vi "Fpga-MicroBlaze-Transmit.vi"(0 "Network API":refnum<class "niInstr Network API FPGA v1.lvclass">, 1 "FIFO In":refnum<k21>, 5 "Controls":T3={"UDP Source Port"=43981, "UDP Destination Port"=61185, "preferred datagram size"=1400, "Use Pattern Gen"=FALSE, "max frame payload"=1472, "minimum packet interval"=1, "stream.num samples 0"=0, "stream.request state 0"=enum."Idle"} {"UDP Destination Port" format="%04x"; "UDP Source Port" format="%04x"}) -> (6 "Indicators":T1)   [LabVIEW 2017, in "My Network FPGA v1.lvlib"]
uses:
  Example SubVIs/My Network FPGA v1.lvlib
  <instrlib>/_niInstr/Network/API/v1/FPGA/niInstr Network API FPGA v1.lvclass
  Example SubVIs/TX Controls.ctl
  <instrlib>/_niInstr/Streaming/v1/Common/Stream State.ctl
  Example SubVIs/TX Indicators.ctl
  <vilib>/rvi/DataTransferAndStorage/Container/Common/niFpgaContainerExecOnDevCompGetState.vi
  <vilib>/rvi/Emulation/niFpgaSctlEmulationGetInTimedLoop.vi
  <vilib>/rvi/errors/niFpgaSetErrorForExecOnDevCompSimple.vi
  <vilib>/rvi/eio/common/nirviEmuReportErrorAndStop.vi
  <vilib>/rvi/interface/RandomDataEmulation/nirviRandomDataAcquireLock.vi
  <vilib>/rvi/interface/RandomDataEmulation/nirviRandomDataQueueStore.vi
  <vilib>/rvi/interface/RandomDataEmulation/nirviRandomDataReleaseLock.vi
  <vilib>/rvi/interface/RandomDataEmulation/nirviFPGAContextMergeError.vi
  <vilib>/rvi/interface/RandomDataEmulation/nirviRandomDataCheckExitLoopConditions.vi
  <vilib>/express/rvi/timingcommon/nirviCommon.vi
  <vilib>/rvi/interface/RandomDataEmulation/niFpgaRandomDataHandleErrors.vi
  <vilib>/rvi/DataTransferAndStorage/Container/XNode/niFpgaContainer.xnode
  <vilib>/rvi/FIFO/Fifo_Resource/niFpgaFifoEmulationRefInMultiElement.vi
  <instrlib>/_niInstr/Network/Ethernet/Utility/v1/FPGA/niInstr Ethernet Utilities FPGA v1.lvlib
  <instrlib>/_niInstr/Streaming/v1/FPGA/niInstr Streaming v1 FPGA.lvlib
  <instrlib>/_niInstr/Streaming/v1/Common/niInstr Streaming v1 Common.lvlib
  <instrlib>/_niInstr/Network/Ethernet/MAC/Raw Stream/v1/niInstr Ethernet MAC Raw Stream v1.lvclass
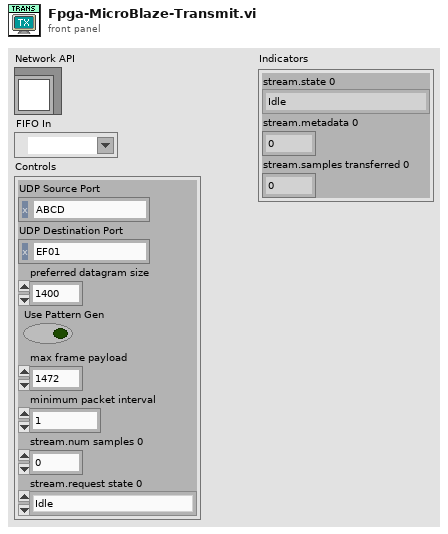
[diagram p1: front panel]
types:
  T1 = typedef "My Network FPGA v1.lvlib/TX Indicators.ctl" = cluster{"stream.state 0":T2, "stream.metadata 0":u64, "stream.samples transferred 0":u64}
  T2 = typedef "niInstr Streaming v1 Common.lvlib/Stream State.ctl" = enum8{"Idle", "Finite Transfer", "Continuous", "Done", "Error", "Not Ready", "Cancel"}
  T3 = typedef "My Network FPGA v1.lvlib/TX Controls.ctl" = cluster{"UDP Source Port":u16, "UDP Destination Port":u16, "preferred datagram size":u16, "Use Pattern Gen":bool, "max frame payload":u16, "minimum packet interval":u32, "stream.num samples 0":u64, "stream.request state 0":T2}
  T4 = cluster{"ready for input (payload data)":bool, "ready for input (start packet)":bool}
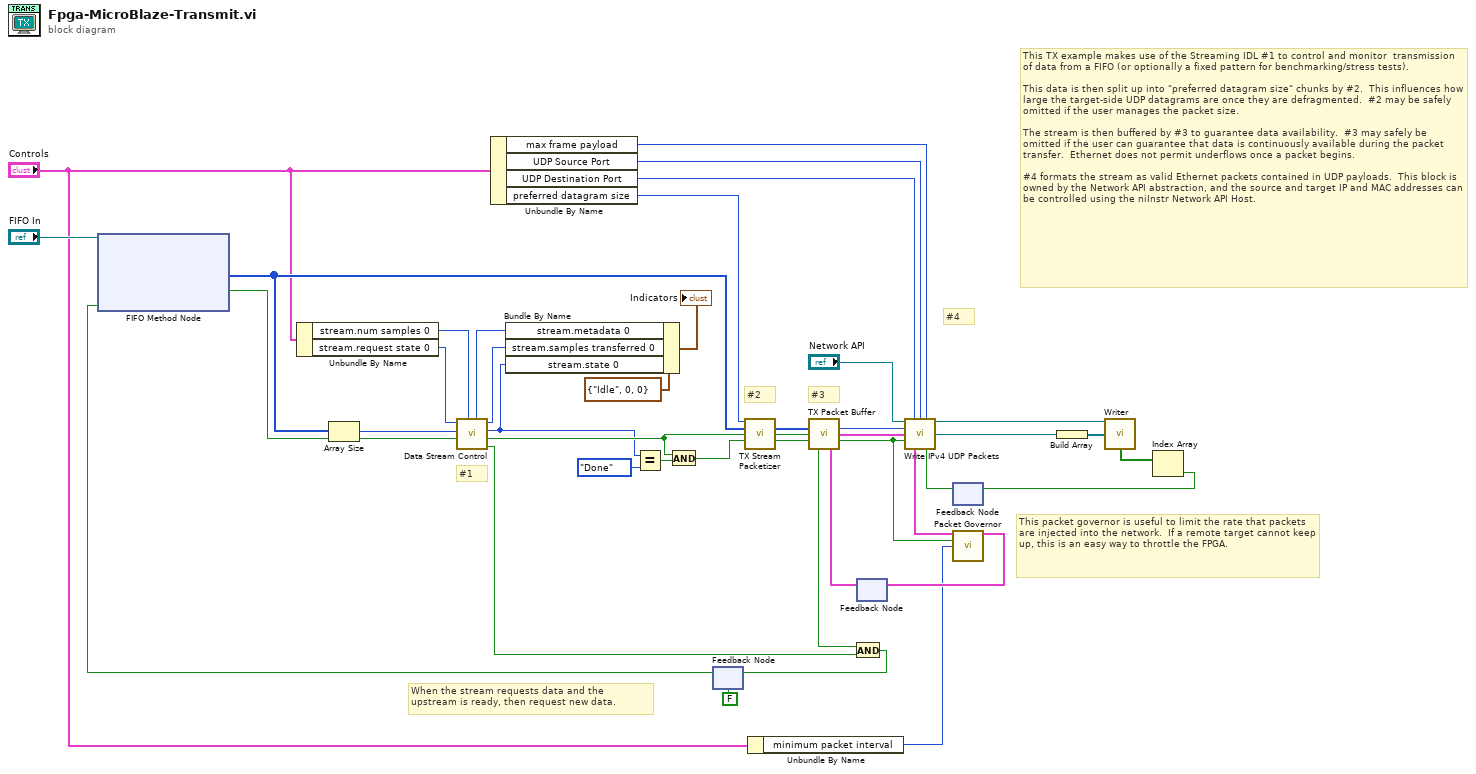
[diagram p0: block diagram]
diagram:
  # "#4"
  # "#3"
  # "#2"
  # "When the stream requests data and the upstream is ready, then request new data."
  # "#1"
  # "This TX example makes use of the Streaming IDL #1 to control and monitor  transmission of data from a FIFO (or optionally a fixed pattern for benchmarking/stress tests).\n\nThis data is then split up into \"preferred datagram size\" chunks by #2.  This influences how large the target-side UDP datagrams are once they are defragmented.  #2 may be safely omitted if the user manages the packet size.\n\nThe stream is then buffered by #3 to guarantee data availability.  #3 may safely be omitted if the user can guarantee that data is continuously available during the packet transfer.  Ethernet does not permit underflows once a packet begins.\n\n#4 formats the stream as valid Ethernet packets contained in UDP payloads.  This block is owned by the Network API abstraction, and the source and target IP and MAC addresses can be controlled using the niInstr Network API Host."
  # "This packet governor is useful to limit the rate that packets are injected into the network.  If a remote target cannot keep up, this is an easy way to throttle the FPGA."
  n1 = Unbundle By Name("Controls") -> ("stream.num samples 0"=w8:u64, "stream.request state 0"=w7:T2)
  n2 = Unbundle By Name("Controls") -> ("max frame payload"=w5:u16, "UDP Source Port"=w4:u16, "UDP Destination Port"=w3:u16, "preferred datagram size"=w6:u16)
  n3 = feedback #1(FALSE ("ready for input")) -> (w34:bool)
  n4 = xnode ("FIFO Method Node")("Ready for Output"=w34, "FIFO In"="FIFO In") -> ("Element"=w21:u8[], "Output Valid"=w33:bool)  [unwired: 1 out]
  n5 = Array Size(array=w21) -> (size(s)=w20:i32)
  n6 = call <instrlib>:"Data Stream Control.vi"("stream.num samples 0"=w8, "data valid"=w33, "element count"=w20, "stream.request state 0"=w7) -> ("request data"=w15:bool, "send data"=w30:bool, "stream.state 0"=w9:T2, "stream.samples transferred 0"=w10:u64, "stream.metadata 0"=w11:u64)  [unwired: 3 in]
  n7 = Bundle By Name(cluster=T1 {"stream.state 0"=enum."Idle", "stream.metadata 0"=0, "stream.samples transferred 0"=0} ("Indicators"), "stream.metadata 0"=w11, "stream.samples transferred 0"=w10, "stream.state 0"=w9) -> (→"Indicators":T1)
  n8 = Equal?(x=w9, y=Stream_State."Done" ("stream.state 0")) -> (x = y?=w31:bool)
  n9 = And(x=w30, y=w31) -> (x .and. y?=w29:bool)
  n10 = call <instrlib>:"TX Stream Packetizer.vi"("preferred datagram size"=w6, "data in"=w21, "data valid in"=w30, "last in"=w29) -> ("data out"=w37:u8[], "data valid out"=w39:bool, "last out"=w38:bool)  [unwired: 8 in, 1 out]
  n11 = Unbundle By Name("Controls") -> ("minimum packet interval"=w1:u32)
  n12 = feedback #2() -> (w35:T4)  [unwired: 1 in]
  n13 = call <instrlib>:"TX Packet Buffer.vi"("data"=w37, "data valid"=w39, "last/flush"=w38, "ready for output?"=w35) -> ("tx bytes to send"=w28:u16, "output data"=w36:cluster{"data":u8[], "data valid":bool}, "start packet"=w17:bool, "ready for input"=w16:bool)  [unwired: 8 in]
  n14 = And(x=w16, y=w15) -> (x .and. y?=w14:bool)
  n15 = feedback-in #1(w14) -> ()
  n16 = feedback #3() -> (w25:bool)  [unwired: 1 in]
  n17 = call <instrlib>:"Write IPv4 UDP Packets.vi"("niInstr Network API FPGA v1.lvclass"="Network API", "UDP destination port"=w3, "UDP source port"=w4, "max frame payload"=w5, "total datagram payload"=w28, "data"=w36, "start packet"=w17, "ready for output"=w25) -> ("niInstr Network API FPGA v1.lvclass out"=w23:refnum<class "niInstr Network API FPGA v1.lvclass">, "niInstr Ethernet MAC Raw Stream v1 out"=w24:refnum<class "niInstr Ethernet MAC Raw Stream v1.lvclass">, "ready for input?"=w18:T4)  [unwired: 5 in]
  n18 = call "Packet Governor.vi"("ready for input? in"=w18, "start packet"=w17, "minimum packet interval"=w1) -> ("ready for input? out"=w19:T4)  [unwired: 12 in]
  n19 = feedback-in #2(w19) -> ()
  n20 = Build Array(w24) -> (w27:refnum<class "niInstr Ethernet MAC Raw Stream v1.lvclass">[])
  n21 = call <instrlib>:"Writer.vi"("niInstr Network API FPGA v1.lvclass"=w23, "input packet streams"=w27) -> ("ready for input"=w26:bool[])  [unwired: 13 in]
  n22 = Index Array(array=w26) -> (element=w40:bool)  [unwired: 1 in]
  n23 = feedback-in #3(w40) -> ()
